vi "Teleop Mode Selector.vi"(8 "Button Cluster":T3, 10 "Drivetrain Command Cluster in":T1) -> (3 "Drivetrain Command Cluster out":T1)   [LabVIEW 2015]
uses:
  Common Code/Gamepads/Button Cluster.ctl
  Drivetrain Commands.ctl
  Drivetrain Modes.ctl
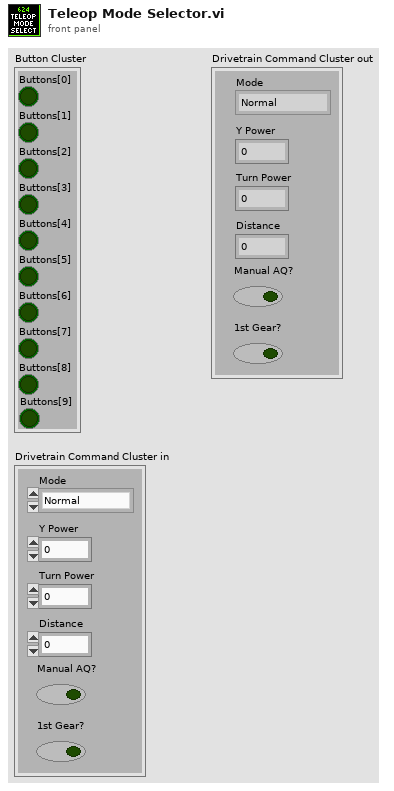
[diagram p1: front panel]
types:
  T1 = typedef "Drivetrain Commands.ctl" = cluster{"Mode":T2, "Y Power":dbl, "Turn Power":dbl, "Distance":sgl, "Manual AQ?":bool, "1st Gear?":bool}
  T2 = typedef "Drivetrain Modes.ctl" = enum16{"Normal", "Cubic Profile", "Trapezoidal Profile", "Turn to Angle", "Distance Drive", "Data Acquisition"}
  T3 = typedef "Button Cluster.ctl" = cluster{"Buttons[0]":bool, "Buttons[1]":bool, "Buttons[2]":bool, "Buttons[3]":bool, "Buttons[4]":bool, "Buttons[5]":bool, "Buttons[6]":bool, "Buttons[7]":bool, "Buttons[8]":bool, "Buttons[9]":bool}
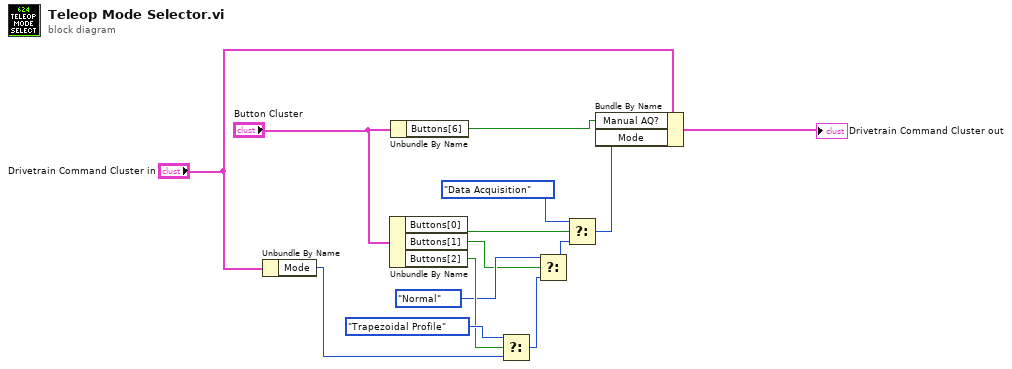
[diagram p0: block diagram]
diagram:
  n1 = Unbundle By Name("Drivetrain Command Cluster in") -> ("Mode"=w1:T2)
  n2 = Unbundle By Name("Button Cluster") -> ("Buttons[0]"=w3:bool, "Buttons[1]"=w5:bool, "Buttons[2]"=w9:bool)
  n3 = Unbundle By Name("Button Cluster") -> ("Buttons[6]"=w12:bool)
  n4 = Select(t=Drivetrain_Modes."Trapezoidal Profile", s=w9, f=w1) -> (s? t:f=w11:T2)
  n5 = Select(t=Drivetrain_Modes."Normal", s=w5, f=w11) -> (s? t:f=w4:T2)
  n6 = Select(t=Drivetrain_Modes."Data Acquisition", s=w3, f=w4) -> (s? t:f=w8:T2)
  n7 = Bundle By Name(cluster="Drivetrain Command Cluster in", "Manual AQ?"=w12, "Mode"=w8) -> (→"Drivetrain Command Cluster out":T1)
